vi "3.1.1-Arbiter.vi"(5 "Joystick Neurons":T1) -> (6 "Inhibit Motors":bool, 8 "Steering Angle, Deg":dbl, 10 "Drive Speed, Mph":dbl, 15 "Lidar Declination, Deg":dbl)   [LabVIEW 2010]
doc: "This VI arbitrates the one command input form the Forebrain, and a set of inputs from the Limbic and Cerrebellum THINK processes and conducts a voting poll arbitor with input from each to determine the one output command.\n\nThis is a voting arbiter, it adds each behaviors vote array, selects maximum (winner) and sends that angle and velocity to the Hindbrain\n\nInputs: 90 cell arrays of weighted direction commands \n\nOutput: Cluster of desried velocity and direction"
uses:
  4-High Neurons/4.6.1-Action Neuron Typedef.ctl
  3.0-Global.vi
panel:
  in  "Hippocampic Neurons":T1
  in  "Neo Cortical Neurons":T1
  in  "Cerebral Neurons":T1
  in  "Limbic Neurons":T1
  in  "Hypo-Thalamal Neurons":T1
  out "Waveform Graph":dbl[][](graph)
  # "This subVI takes the three\nACT commands; one from the forebrain \nand three from the Midbrain and\naverages them"
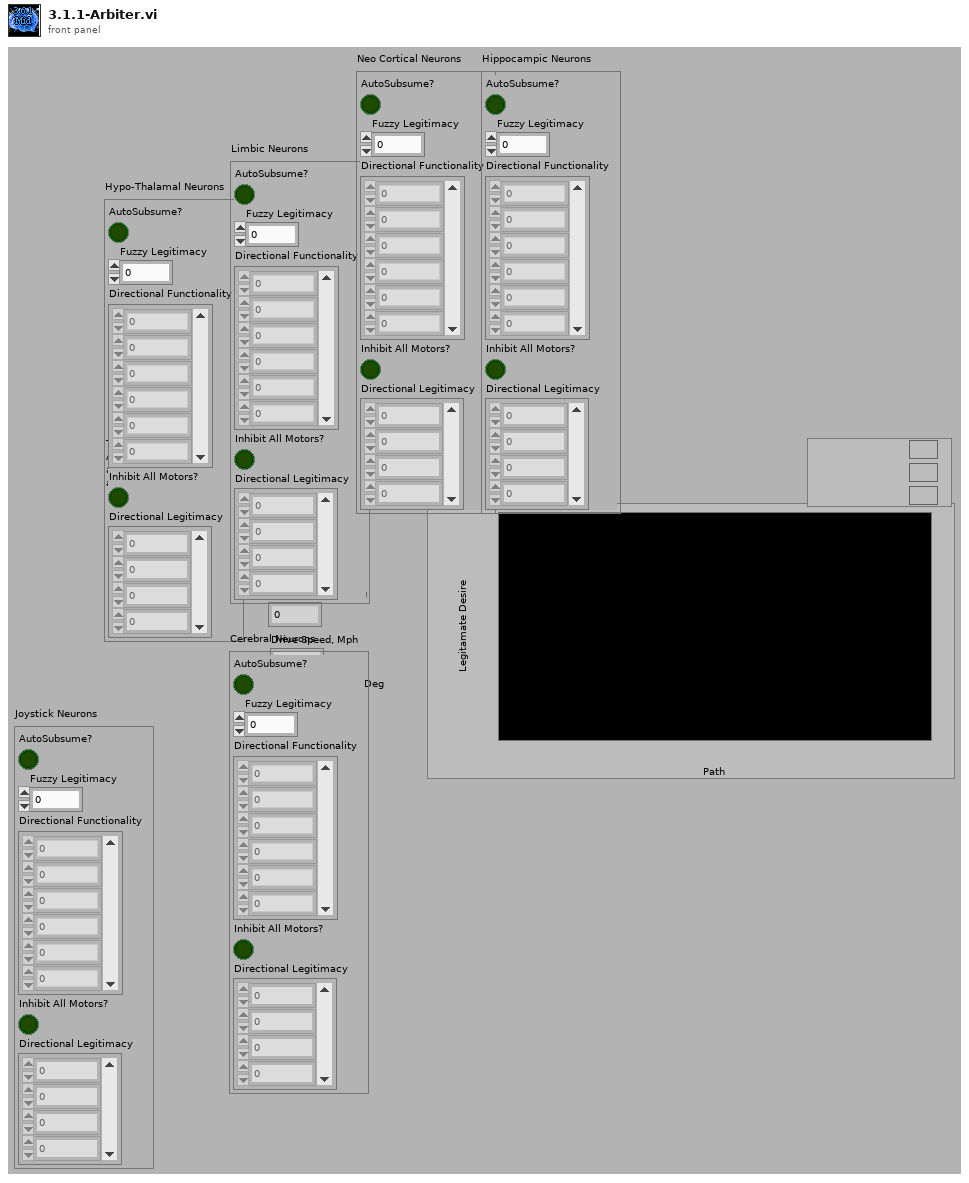
[diagram p1: front panel]
types:
  T1 = typedef "4.6.1-Action Neuron Typedef.ctl" = cluster{"AutoSubsume?":bool, "Fuzzy Legitimacy":dbl, "Directional Functionality":dbl[], "Inhibit All Motors?":bool, "Directional Legitimacy":u8[]}
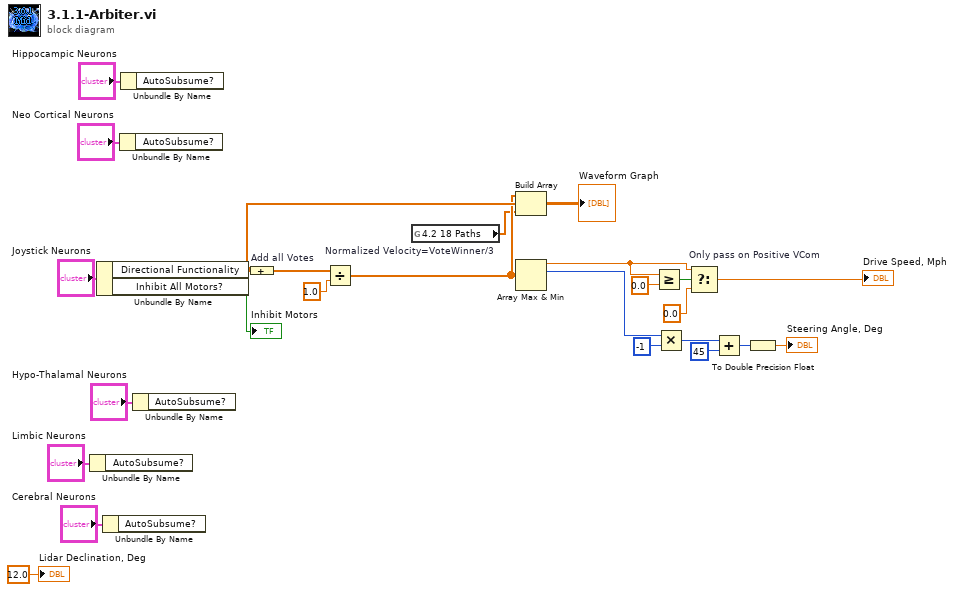
[diagram p0: block diagram]
diagram:
  n1 = Unbundle By Name("Limbic Neurons") -> ()  [unwired: 1 out]
  n2 = Unbundle By Name("Joystick Neurons") -> ("Directional Functionality"=w7:dbl[], "Inhibit All Motors?"=→"Inhibit Motors":bool)
  n3 = Unbundle By Name("Cerebral Neurons") -> ()  [unwired: 1 out]
  n4 = Unbundle By Name("Neo Cortical Neurons") -> ()  [unwired: 1 out]
  n5 = Unbundle By Name("Hippocampic Neurons") -> ()  [unwired: 1 out]
  n6 = Unbundle By Name("Hypo-Thalamal Neurons") -> ()  [unwired: 1 out]
  n7 = Compound Arithmetic op=ADD "Add all Votes"(w7) -> (w19:dbl[])
  n8 = Divide "Normalized Velocity=VoteWinner/3"(x=w19, y=1.0) -> (x/y=w6:dbl[])
  n9 = global read "3.0-Global.vi" "4.2 18 Paths"() -> (w1:dbl[])
  n10 = Build Array "Build Array"(w6, w7, w1) -> (→"Waveform Graph":dbl[][])
  n11 = Array Max & Min(array=w6) -> (max value=w15:dbl, max index (indices)=w25:i32)  [unwired: 2 out]
  n12 = Greater Or Equal?(x=w15, y=0.0) -> (x >= y?=w16:bool)
  n13 = Multiply(x=w25, y=-1) -> (x*y=w23:i32)
  n14 = Select "Only pass on Positive VCom"(t=w15, s=w16, f=0.0) -> (s? t:f=→"Drive Speed, Mph":dbl)
  n15 = Add(x=w23, y=45) -> (x+y=w21:i32)
  n16 = To Double Precision Float(number=w21) -> (double precision float=→"Steering Angle, Deg":dbl)
  "Lidar Declination, Deg" <- 12.0 ("Lidar Declination, Deg")
